vi "Remove Step at Index.vi"(8 "error in (no error)":errorcluster, 10 "Index":i32, 11 "Sequence in":refnum<class "Sequence.lvclass">) -> (0 "error out":errorcluster, 3 "Sequence out":refnum<class "Sequence.lvclass">)   [LabVIEW 2024, in "Ramses Sequencer.lvlib" / "Sequence.lvclass"]
uses:
  Sequence.lvclass
  Sequence.lvclass/Sequence.ctl
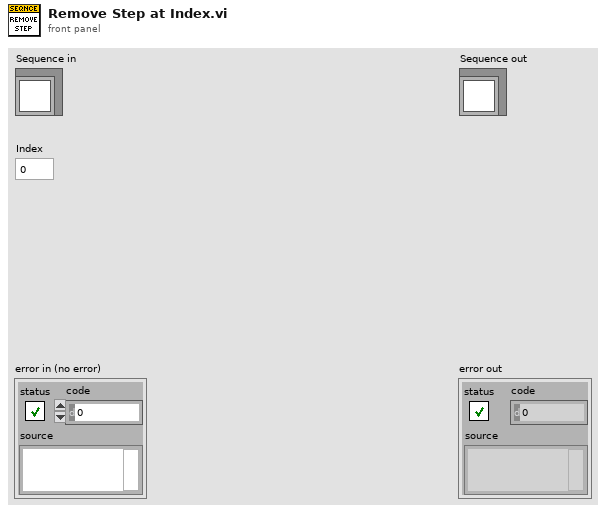
[diagram p1: front panel]
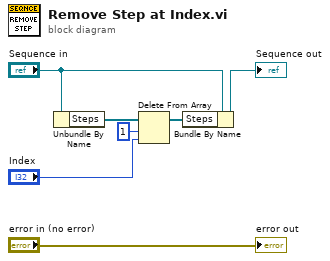
[diagram p0: block diagram]
diagram:
  n1 = Unbundle By Name("Sequence in") -> ("Steps"=w4:refnum<class "Base Step.lvclass">[])
  n2 = Delete From Array(array=w4, length=1, index="Index") -> (array with subset deleted=w3:refnum<class "Base Step.lvclass">[])  [unwired: 1 out]
  n3 = Bundle By Name(cluster="Sequence in", "Steps"=w3) -> (→"Sequence out":refnum<class "Sequence.lvclass">)
  "error out" <- "error in (no error)"
